vi "connect bundle and subvi.vi"(8 "error in":errorcluster, 9 "Unbundle ref in":refnum<vi>, 10 "Bundle ref in":refnum<vi>, 11 "SubVI in":refnum<vi>) -> (0 "error out":errorcluster)   [LabVIEW 2013]
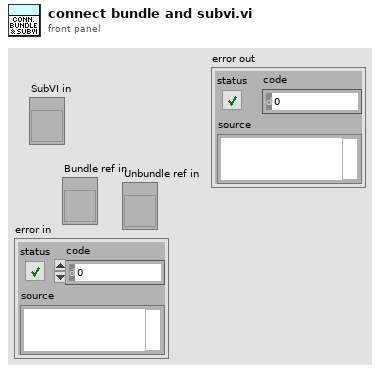
[diagram p1: front panel]
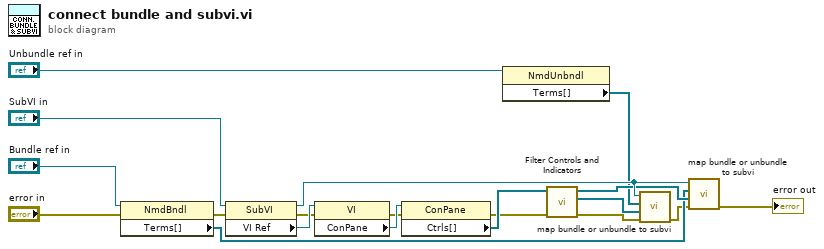
[diagram p0: block diagram]
diagram:
  n1 = property class="NmdBndl"(reference="Bundle ref in", error in="error in") -> (error out=w15:errorcluster, "Terms[]"=w5:refnum<vi>[])  [unwired: 1 out]
  n2 = property class="SubVI"(reference="SubVI in", error in=w15) -> (reference out=w8:refnum<vi>, error out=w14:errorcluster, "VI Ref"=w18:refnum<vi>)
  n3 = property class="VI"(reference=w18, error in=w14) -> (error out=w13:errorcluster, "ConPane"=w19:refnum<vi>)  [unwired: 1 out]
  n4 = property class="ConPane"(reference=w19, error in=w13) -> (error out=w3:errorcluster, "Ctrls[]"=w11:refnum<vi>[])  [unwired: 1 out]
  n5 = property class="NmdUnbndl"(reference="Unbundle ref in") -> ("Terms[]"=w6:refnum<vi>[])  [unwired: 1 in, 2 out]
  n6 = call "Filter Controls and Indicators.vi"("error in"=w3, "Ctrls[]"=w11) -> ("error out"=w2:errorcluster, "Controls"=w9:refnum<vi>[], "Indicators"=w7:refnum<vi>[])  [unwired: 7 in]
  n7 = call "map bundle or unbundle to subvi.vi"("error in (no error)"=w2, "Controls/Indicators"=w9, "Terms[]"=w6, "SubVI in"=w8) -> ("error out"=w4:errorcluster)  [unwired: 7 in]
  n8 = call "map bundle or unbundle to subvi.vi"("error in (no error)"=w4, "Controls/Indicators"=w7, "Terms[]"=w5, "SubVI in"=w8) -> ("error out"=→"error out":errorcluster)  [unwired: 7 in]
